vi "LVClass_HasoSlopes Apply Modulator.vi"(0 "HasoSlopes in":refnum<class "HasoSlopes.lvclass">, 7 "filter":T1, 11 "error in (no error)":errorcluster) -> (4 "HasoSlopes out":refnum<class "HasoSlopes.lvclass">, 15 "error out":errorcluster)   [LabVIEW 2020, in "HasoSlopes.lvclass"]
uses:
  HasoSlopes.lvclass
  Controls/SlopesPostProcessorList - Modulator.ctl
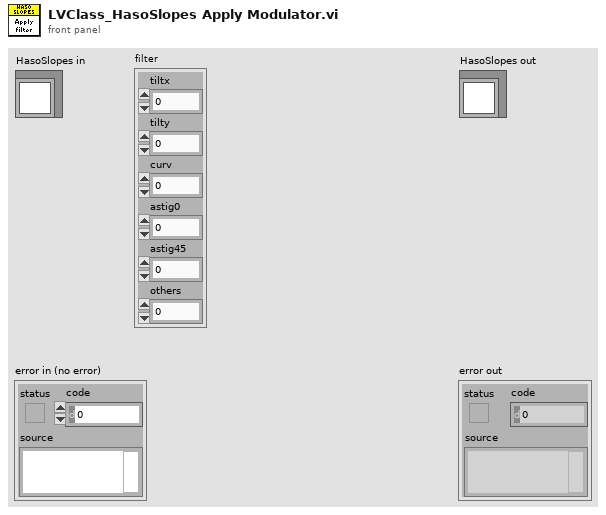
[diagram p1: front panel]
types:
  T1 = typedef "SlopesPostProcessorList - Modulator.ctl" = cluster{"tiltx":sgl, "tilty":sgl, "curv":sgl, "astig0":sgl, "astig45":sgl, "others":sgl}
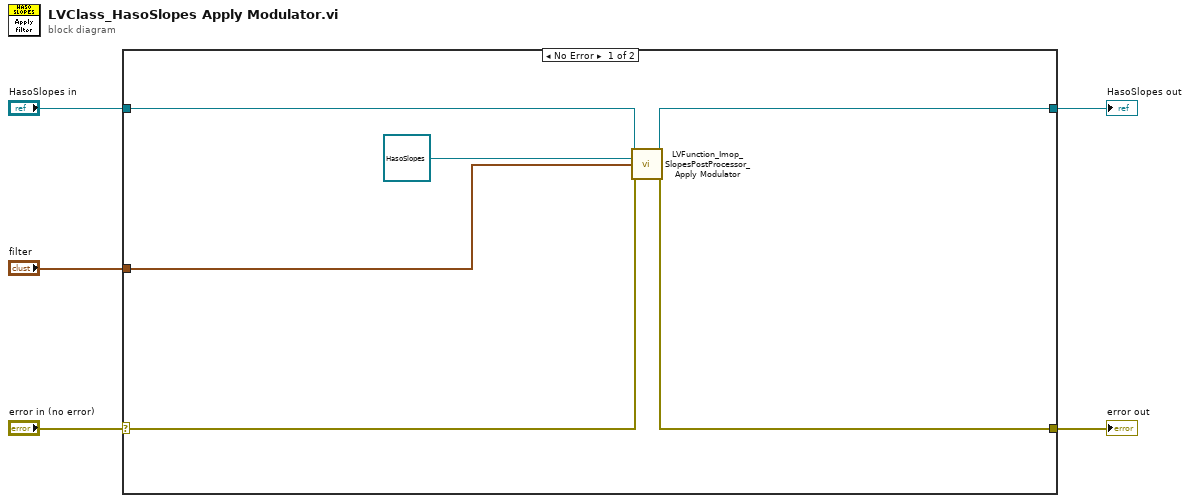
[diagram p0: block diagram]
diagram:
  n1 = case shown="No Error" "error in (no error)" {
    selector: "error in (no error)" -> [w10 w13]
    tunnel: [w9 w13] -> w3
    tunnel: [w7 w12] -> w4
    tunnel: "HasoSlopes in" -> [w8 w12]
    tunnel: "filter" -> [w11 _]
    frame No Error {
      n2 = call "LVFunction_Imop_SlopesPostProcessor_Apply Modulator.vi"("HasoSlopes in"=w8, "HasoSlopes OUT"=refnum<class "HasoSlopes.lvclass"> refnum, "filter"=w11, "error in (no error)"=w10) -> ("HasoSlopes out"=w7:refnum<class "HasoSlopes.lvclass">, "error out"=w9:errorcluster)  [unwired: 9 in, 1 out]
    }
    frame Error {
    }
  }
  "error out" <- w3
  "HasoSlopes out" <- w4
